vi "Write TCPClient.vi"(8 "error in (no error)":errorcluster, 10 "TCPClient":refnum<class "TCPClient.lvclass">, 11 "SpectrographClientCommunicator in":refnum<class "SpectrographClientCommunicator.lvclass">) -> (0 "error out":errorcluster, 3 "SpectrographClientCommunicator out":refnum<class "SpectrographClientCommunicator.lvclass">)   [LabVIEW 2016, in "SpectrographClientCommunicator.lvclass"]
uses:
  SpectrographClientCommunicator.lvclass
  ts_labview_tcp/TCPClient/TCPClient.lvclass
  SpectrographClientCommunicator.lvclass/SpectrographClientCommunicator.ctl
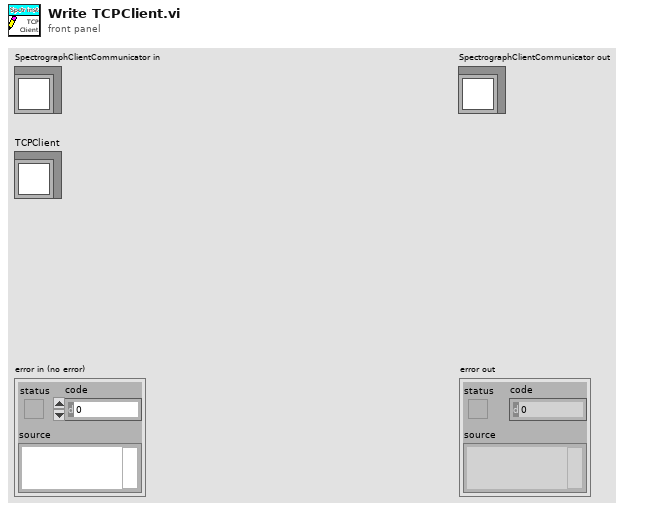
[diagram p1: front panel]
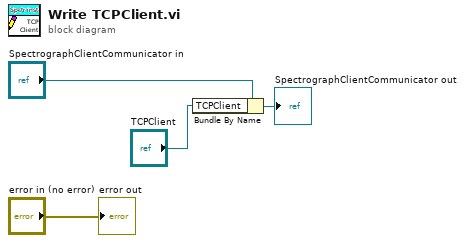
[diagram p0: block diagram]
diagram:
  n1 = Bundle By Name(cluster="SpectrographClientCommunicator in", "TCPClient"="TCPClient") -> (→"SpectrographClientCommunicator out":refnum<class "SpectrographClientCommunicator.lvclass">)
  "error out" <- "error in (no error)"
